vi "PopElement.vi"(8 "error in (no error)":errorcluster, 11 "Astar Open List in":refnum<class "NI_Robotics_Priority Queue.lvclass">) -> (0 "error out":errorcluster, 1 "empty":bool, 2 "open list element":T1, 3 "Astar Open List out":refnum<class "NI_Robotics_Priority Queue.lvclass">)   [LabVIEW 2017, in "NI_Robotics_Priority Queue.lvclass"]
uses:
  <vilib>/robotics/Navigation/shared/Priority Queue/NI_Robotics_Priority Queue.lvclass
  <vilib>/robotics/Navigation/shared/Priority Queue/Open List Element.ctl
  <vilib>/robotics/Navigation/shared/MapNode/AbstractMapNode/NI_Robotics_AbstractMapNode.lvclass
  <vilib>/robotics/Navigation/shared/Priority Queue/NI_Robotics_Priority Queue.lvclass/NI_Robotics_Priority Queue.ctl
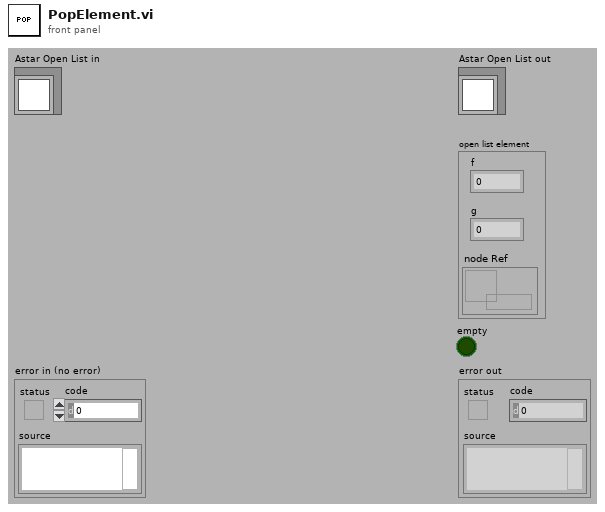
[diagram p1: front panel]
types:
  T1 = typedef "NI_Robotics_Priority Queue.lvclass/Open List Element.ctl" = cluster{"f":dbl, "g":dbl, "node Ref":refnum<data-value>}
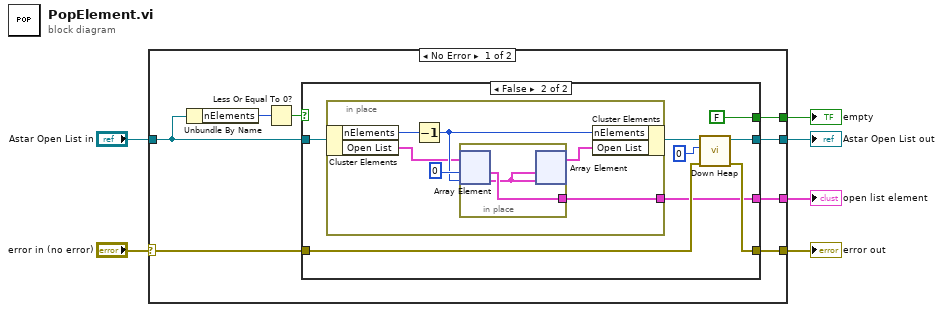
[diagram p0: block diagram]
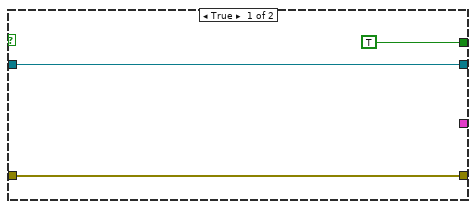
[diagram p2: hidden frame]
diagram:
  n1 = case shown="No Error" "error in (no error)" {
    selector: "error in (no error)" -> [w9 w35]
    tunnel: [w14 w35] -> w6
    tunnel: [w13 w34] -> w5
    tunnel: "Astar Open List in" -> [w12 w34]
    tunnel: [w11 _] -> w3
    tunnel: [w10 _] -> w2
    frame No Error {
      n2 = Unbundle By Name(w12) -> ("nElements"=w8:i32)
      n3 = Less Or Equal To 0?(x=w8) -> (x <= 0?=w7:bool)
      n4 = case shown="False" w7 {
        tunnel: [w16 w21] -> w14
        tunnel: [w17 w23] -> w13
        tunnel: w12 -> [w17 w25]
        tunnel: w9 -> [w16 w22]
        tunnel: [_ w19] -> w11
        tunnel: [TRUE ("status") FALSE ("status")] -> w10
        frame True {
        }
        frame False {
          n5 = in-place {
            in-place-border: [w26] -> w19
            n6 = in-place-cluster #1(w25) -> ("nElements"=w31:i32, "Open List"=w28:T1[])
            n7 = Decrement(x=w31) -> (x-1=w29:i32)
            n8 = in-place {
              in-place-border: [w33] -> w26
              n9 = in-place-array #2(w28, 0 ("index"), w29) -> (w33:T1, w32:T1)
              n10 = in-place-array #2(w32, w32) -> (w27:T1[])  [unwired: 2 out]
            }
            n11 = in-place-cluster #1("nElements"=w29, "Open List"=w27) -> (w24:refnum<class "NI_Robotics_Priority Queue.lvclass">)
          }
          n12 = call <vilib>:"Down Heap.vi"("error in (no error)"=w22, "index"=0, "Astar Open List in"=w24) -> ("error out"=w21:errorcluster, "Astar Open List out"=w23:refnum<class "NI_Robotics_Priority Queue.lvclass">)  [unwired: 7 out]
        }
      }
    }
    frame Error {
    }
  }
  "error out" <- w6
  "Astar Open List out" <- w5
  "open list element" <- w3
  "empty" <- w2
